vi "saveXMLFile.vi"(8 "error in (no error)":errorcluster, 9 "xmlString":string="xmlString", 11 "XmlParser in":refnum<class "XmlParser.lvclass">) -> (0 "error out":errorcluster, 3 "XmlParser out":refnum<class "XmlParser.lvclass">)   [LabVIEW 2011, in "Tools.lvlib" / "xml.lvlib" / "XmlParser.lvclass"]
doc: "Save xml string to document"
uses:
  XmlParser.lvclass
  XmlParser.lvclass/XmlParser.ctl
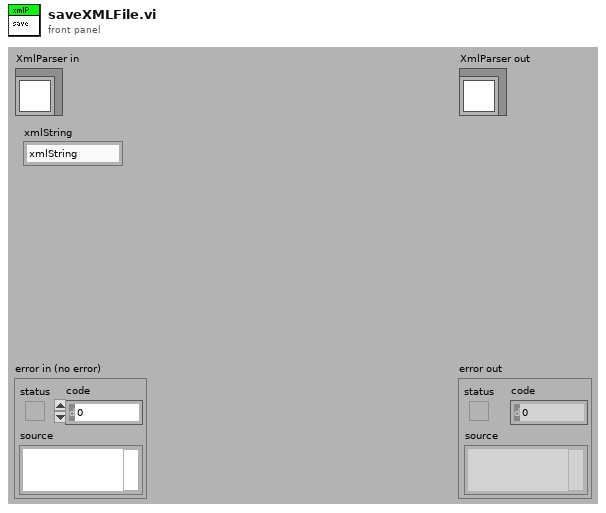
[diagram p1: front panel]
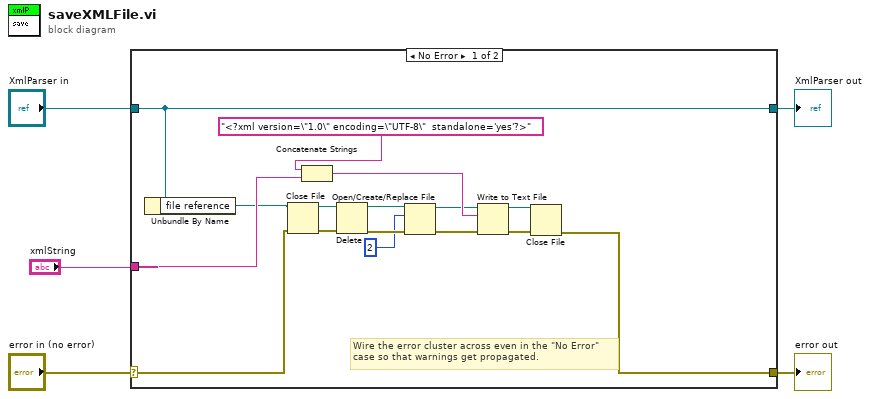
[diagram p0: block diagram]
diagram:
  n1 = case shown="No Error" "error in (no error)" {
    selector: "error in (no error)" -> [w12 w23]
    tunnel: [w19 w23] -> w4
    tunnel: [w15 w22] -> w2
    tunnel: "XmlParser in" -> [w15 w22]
    tunnel: "xmlString" -> [w16 _]
    frame No Error {
      # "Wire the error cluster across even in the \"No Error\"\ncase so that warnings get propagated."
      n2 = Unbundle By Name(w15) -> ("file reference"=w13:refnum<file>)
      n3 = Close File(refnum=w13, error in=w12) -> (path=w11:path, error out=w10:errorcluster)
      n4 = Concatenate Strings("<?xml version=\"1.0\" encoding=\"UTF-8\"  standalone='yes'?>", w16) -> (w18:string)
      n5 = Delete(path (use dialog)=w11, error in=w10) -> (deleted path=w9:path, error out=w8:errorcluster)  [unwired: 3 in, 1 out]
      n6 = Open/Create/Replace File(file path (use dialog)=w9, error in=w8, operation (0:open)=2) -> (refnum out=w14:refnum<file>, error out=w7:errorcluster)  [unwired: 3 in, 1 out]
      n7 = Write to Text File(file (use dialog)=w14, text=w18, error in=w7) -> (refnum out=w21:refnum<file>, error out=w20:errorcluster)  [unwired: 1 in, 1 out]
      n8 = Close File(refnum=w21, error in=w20) -> (error out=w19:errorcluster)  [unwired: 1 out]
    }
    frame Error {
    }
  }
  "error out" <- w4
  "XmlParser out" <- w2
